vi "PH_PILS.vis ResetExtEOKnob.vi"(0 "i ref in":refnum<vi>, 5 "error IO":errorcluster) -> (14 "i ref out":refnum<vi>, 19 "error out":errorcluster)   [LabVIEW 2014, in "PH_PILS.lvlib"]
uses:
  PH_PILS.lvlib
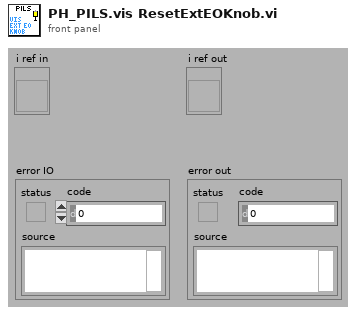
[diagram p1: front panel]
types:
  T1 = typedef "PH_PILS.lvlib/PH_PILS.i attribute.ctl" = cluster{"Boolean":cluster{"GUI Ref":refnum<vi>, "Status":i32}[], "GUI Refs Exp. Shutters":cluster{"1":refnum<vi>, "2":refnum<vi>, "3":refnum<vi>, "4":refnum<vi>}, "Tristate2Run GUI Refs":refnum<vi>[], "EO-Likes":cluster{"GUI Ref":refnum<vi>, "Status":i32}[], "Operation Mode":cluster{"Operation Mode":T2, "GUI":cluster{"Ref State":refnum<vi>, "Ref":refnum<vi>}, "Servicemode":cluster{"Tagname":string, "Status":i32}, "Labormode":cluster{"Tagname":string, "Status":i32}, "Searchmode":cluster{"Tagname":string, "Status":i32}, "Shotmode":cluster{"Tagname":string, "Status":i32}}, "Submode":cluster{"Submode":T3, "GUI":cluster{"Ref State":refnum<vi>, "Ref":refnum<vi>}, "Submode":cluster{"Tagname":string, "Status":i32}}, "Experiment":cluster{"Experiment":enum16{"unknown", "intern", "4 (Z6)", "3", "2", "1"}, "GUI":cluster{"Ref State":refnum<vi>, "Ref":refnum<vi>}, "intern":cluster{"Tagname":string, "Status":i32}, "Exp 4":cluster{"Tagname":string, "Status":i32}, "Exp 3":cluster{"Tagname":string, "Status":i32}, "Exp 2":cluster{"Tagname":string, "Status":i32}, "Exp 1":cluster{"Tagname":string, "Status":i32}}, "TristateNormal":cluster{"GUI Ref":refnum<vi>, "Status":i32}[], "Door Tags":cluster{"GUI Ref":refnum<vi>, "Status":i32}[], "GUIlessTags":cluster{"Name":string, "Status":i32}[], "Beamline GUI Refs":refnum<vi>[], "Special Boolean":cluster{"GUI Ref":refnum<vi>, "Status":i32}[], "Laserpower":cluster{"GUI Ref":refnum<vi>, "Status":i32}[], "Shutter":cluster{"GUI Ref":refnum<vi>, "Status":i32}[], "Tristate EO Like":cluster{"GUI Ref":refnum<vi>, "Status":i32}[], "PP":cluster{"GUI Ref":refnum<vi>, "Status":i32, "Head Ref":refnum<vi>, "Slider Ref":refnum<vi>}[], "Switch Knobs":cluster{"GUI Ref":refnum<vi>, "Status":i32}[], "Latch Knob GUI Refs":refnum<vi>[], "FailureCounter":i32, "Enabled Status":cluster{"Laser":i32, "PreAmp":i32, "MainAmp":i32}, "Mercury":refnum<vi>, "Instance Rods":string, "Logfile":path, "Beckhoff-Instance Internal":string, "Beckhoff-Instance External":string, "Enabling Rights":cluster{"Name":string, "Password":string, "PA?":bool, "MA?":bool, "Exp?":bool}[]}
  T2 = typedef "PH_PILS.lvlib/PH_PILS.Operation Mode.ctl" = enum16{"unknown", "Service", "Labor", "Search", "Shot"}
  T3 = typedef "PH_PILS.lvlib/PH_PILS.Submode.ctl" = enum16{"unknown", "HV-Normal", "HV-Test"}
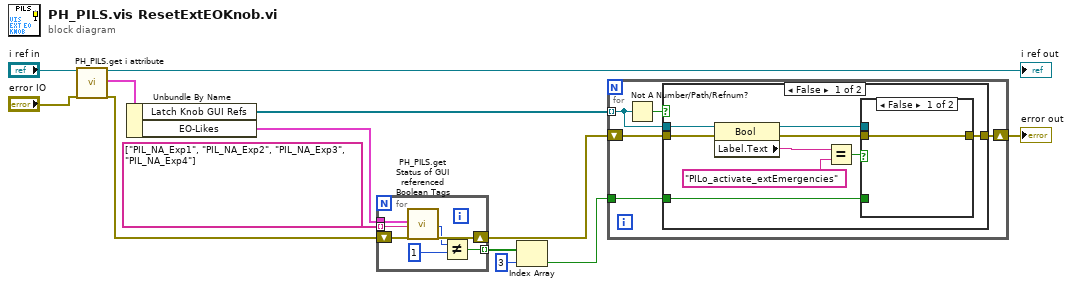
[diagram p0: block diagram]
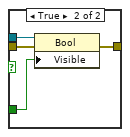
[diagram p2: hidden frame]
diagram:
  n1 = call "PH_PILS.get i attribute.vi"("i ref in"="i ref in", "error in (no error)"="error IO") -> ("i ref out"=→"i ref out":refnum<vi>, "i attribute"=w10:T1, "error out"=w6:errorcluster)  [unwired: 15 in]
  n2 = Unbundle By Name(w10) -> ("Latch Knob GUI Refs"=w1:refnum<vi>[], "EO-Likes"=w8:cluster{"GUI Ref":refnum<vi>, "Status":i32}[])
  n3 = for {
    tunnel: w8 -> [w19]
    shift-right: [w20] -> w2
    shift-left: w6 -> [w17]
    tunnel: string[] ["PIL_NA_Exp1", "PIL_NA_Exp2", "PIL_NA_Exp3", "PIL_NA_Exp4"] -> [w18] mode=indexing
    tunnel: [w16] -> w5 mode=indexing
    n4 = call "PH_PILS.get Status of GUI referenced Boolean Tags.vi"("Tags"=w19, "Tagname"=w18, "error in"=w17) -> ("Status"=w15:i32, "error out"=w20:errorcluster)  [unwired: 13 in, 2 out]
    n5 = Not Equal?(x=w15, y=1) -> (x != y?=w16:bool)
  }
  n6 = Index Array(array=w5, index=3) -> (element=w4:bool)
  n7 = for {
    tunnel: w4 -> [w23]
    shift-right: [w24] -> w9
    shift-left: w2 -> [w22]
    tunnel: w1 -> [w21] mode=indexing
    n8 = Not A Number/Path/Refnum?(number/path/refnum=w21) -> (NaN/Path/Refnum?=w25:bool)
    n9 = case shown="False" w25 {
      tunnel: w22 -> [w32 w40]
      tunnel: w21 -> [w30 _]
      tunnel: [w34 w40] -> w24
      tunnel: w23 -> [w33 _]
      frame False {
        n10 = property class="Bool"(reference=w30, error in=w32) -> (reference out=w29:refnum<vi>, error out=w31:errorcluster, "Label.Text"=w28:string)
        n11 = Equal?(x=w28, y="PILo_activate_extEmergencies") -> (x = y?=w26:bool)
        n12 = case shown="False" w26 {
          tunnel: [w35 w39] -> w34
          tunnel: w33 -> [_ w38]
          tunnel: w31 -> [w35 w37]
          tunnel: w29 -> [_ w36]
          frame False {
          }
          frame True {
            n13 = property class="Bool"(reference=w36, error in=w37, "Visible"=w38) -> (error out=w39:errorcluster)  [unwired: 1 out]
          }
        }
      }
      frame True {
      }
    }
  }
  "error out" <- w9
